vi "FunctDataMgr.Update Result Table Value.vi"(8 "error in (no error)":errorcluster, 11 "FunctDataMgr in":refnum<class "FunctDataMgr.lvclass">) -> (0 "error out":errorcluster, 3 "FunctDataMgr out":refnum<class "FunctDataMgr.lvclass">)   [LabVIEW 2018, in "FunctDataMgr.lvclass"]
uses:
  FunctDataMgr.lvclass
  FunctDataMgr.lvclass/FunctDataMgr.ctl
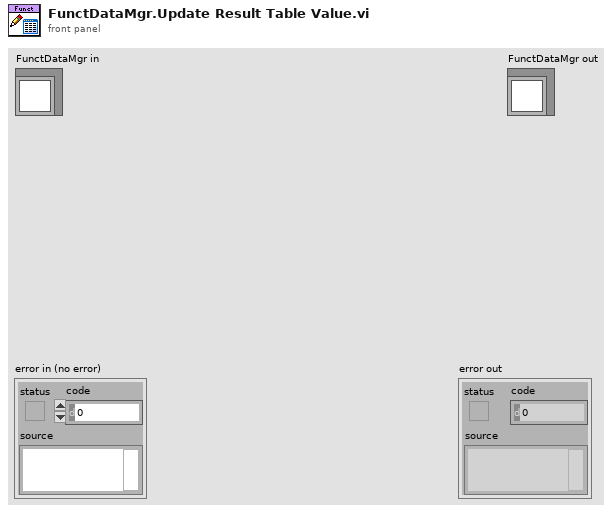
[diagram p1: front panel]
types:
  T1 = typedef "Report.Result FileDataObject.ctl" = cluster{"Cnt":i32, "Step":string, "Category":string, "Name":string, "Type":string, "File Name":string, "Time":string, "Path":path}
  T2 = typedef "Result.Numeric.ctl" = cluster{"Cnt":i32, "Step":string, "Category":string, "Name":string, "Value":dbl, "Units":string, "LimType":T3, "LL":dbl, "UL":dbl, "Status":T4, "Code":i32, "Desc":string, "Time":timestamp}
  T3 = typedef "Result.Limit Type.ctl" = enum16{"None", "EQ", "NE", "GT", "LT", "GE", "LE", "GTLT", "GELE", "GELT", "GTLE", "LTGT", "LEGE", "LEGT", "LTGE", "Contains", "NotContains"}
  T4 = typedef "Result.Measurement and Attribute Item Status.ctl" = i32
  T5 = typedef "Result.Attribute.ctl" = cluster{"Cnt":i32, "Step":string, "Category":string, "Name":string, "Value":string, "Status":T4, "Code":i32, "Desc":string, "Time":timestamp}
  T6 = typedef "Result.Measurement Item.ctl" = cluster{"Cnt":i32, "Step":string, "Category":string, "Name":string, "Value":string, "Units":string, "LimType":string, "LL":string, "UL":string, "Status":T4, "Code":i32, "Desc":string, "Time":timestamp}
  T7 = typedef "Result.Results Table Record.ctl" = cluster{"Cnt":i32, "Step":string, "Category":string, "Name":string, "Value":string, "Units":string, "LimType":string, "LL":string, "UL":string, "Status":string, "Status Color":u32, "Code":i32, "Desc":string}
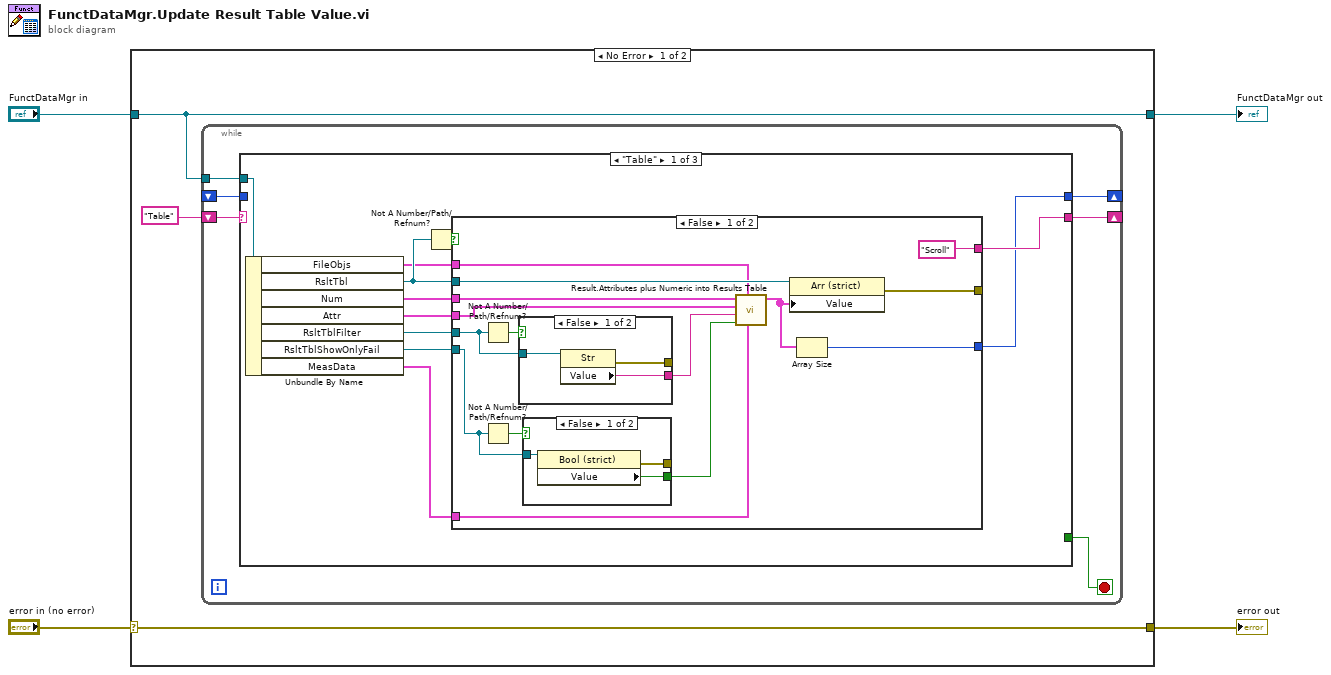
[diagram p0: block diagram]
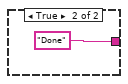
[diagram p4: hidden frame]
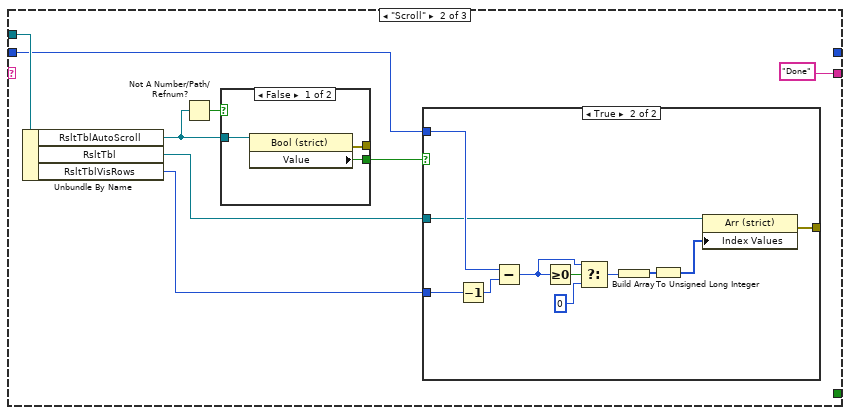
[diagram p5: hidden frame]
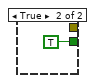
[diagram p7: hidden frame]
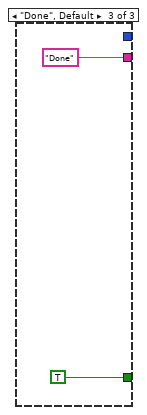
[diagram p8: hidden frame]
diagram:
  n1 = case shown="No Error" "error in (no error)" {
    selector: "error in (no error)" -> [w7 w73]
    tunnel: [w7 w73] -> w3
    tunnel: [w6 w72] -> w1
    tunnel: "FunctDataMgr in" -> [w6 w72]
    frame No Error {
      n2 = while {
        tunnel: w6 -> [w13]
        shift-right: [w10] -> _
        shift-left: "Table" -> [w12]
        shift-right: [w9] -> _
        shift-left: _ -> [w8]
        stop <- w11 stop-if-true
        n3 = case shown="\"Table\"" w12 {
          tunnel: w13 -> [w24 w54 _]
          tunnel: [_ _ TRUE] -> w11
          tunnel: [w21 "Done" "Done"] -> w10
          tunnel: [w16 _ _] -> w9
          tunnel: w8 -> [_ w50 _]
          frame "Table" {
            n4 = Unbundle By Name(w24) -> ("FileObjs"=w14:T1[], "RsltTbl"=w23:refnum<vi>, "Num"=w20:T2[], "Attr"=w19:T5[], "RsltTblFilter"=w18:refnum<vi>, "RsltTblShowOnlyFail"=w17:refnum<vi>, "MeasData"=w15:T6[])
            n5 = Not A Number/Path/Refnum?(number/path/refnum=w23) -> (NaN/Path/Refnum?=w22:bool)
            n6 = case shown="False" w22 {
              tunnel: w23 -> [w39 _]
              tunnel: [w38 _] -> _
              tunnel: ["Scroll" "Done"] -> w21
              tunnel: w20 -> [w36 _]
              tunnel: w19 -> [w35 _]
              tunnel: w18 -> [w34 _]
              tunnel: w17 -> [w30 _]
              tunnel: [w27 _] -> w16
              tunnel: w15 -> [w26 _]
              tunnel: w14 -> [w25 _]
              frame False {
                n7 = Not A Number/Path/Refnum?(number/path/refnum=w34) -> (NaN/Path/Refnum?=w33:bool)
                n8 = Not A Number/Path/Refnum?(number/path/refnum=w30) -> (NaN/Path/Refnum?=w31:bool)
                n9 = case shown="False" w33 {
                  tunnel: w34 -> [w45 _]
                  tunnel: [w44 _] -> _
                  tunnel: [w43 _] -> w32
                  frame False {
                    n10 = property class="Str"(reference=w45) -> (error out=w44:errorcluster, "Value"=w43:string)  [unwired: 1 in, 1 out]
                  }
                  frame True {
                  }
                }
                n11 = case shown="False" w31 {
                  tunnel: w30 -> [w42 _]
                  tunnel: [w41 _] -> _
                  tunnel: [w40 _] -> w29
                  frame False {
                    n12 = property class="Bool (strict)"(reference=w42) -> (error out=w41:errorcluster, "Value"=w40:bool)  [unwired: 1 in, 1 out]
                  }
                  frame True {
                  }
                }
                n13 = call "Result.Attributes plus Numeric into Results Table.vi"("Meas"=w26, "File Data Objs"=w25, "Show Only Failures"=w29, "Filter"=w32, "Attribute Data"=w35, "Numeric Data"=w36) -> ("Results Table"=w28:T7[])  [unwired: 5 in]
                n14 = property class="Arr (strict)"(reference=w39, "Value"=w28) -> (error out=w38:errorcluster)  [unwired: 1 in, 1 out]
                n15 = Array Size(array=w28) -> (size(s)=w27:i32)
              }
              frame True {
              }
            }
          }
          frame "Scroll" {
            n16 = Unbundle By Name(w54) -> ("RsltTblAutoScroll"=w53:refnum<vi>, "RsltTbl"=w47:refnum<vi>, "RsltTblVisRows"=w48:i32)
            n17 = Not A Number/Path/Refnum?(number/path/refnum=w53) -> (NaN/Path/Refnum?=w52:bool)
            n18 = case shown="False" w52 {
              tunnel: w53 -> [w68 _]
              tunnel: [w67 TRUE] -> w49
              tunnel: [w66 _] -> _
              frame False {
                n19 = property class="Bool (strict)"(reference=w68) -> (error out=w66:errorcluster, "Value"=w67:bool)  [unwired: 1 in, 1 out]
              }
              frame True {
              }
            }
            n20 = case shown="True" w49 {
              tunnel: w50 -> [_ w60]
              tunnel: w48 -> [_ w59]
              tunnel: w47 -> [_ w58]
              tunnel: [_ w56] -> _
              frame False {
              }
              frame True {
                n21 = Decrement(x=w59) -> (x-1=w61:i32)
                n22 = Subtract(x=w60, y=w61) -> (x-y=w55:i32)
                n23 = Greater Or Equal To 0?(x=w55) -> (x >= 0?=w62:bool)
                n24 = Select(t=w55, s=w62, f=0) -> (s? t:f=w64:i32)
                n25 = Build Array(w64) -> (w65:i32[])
                n26 = To Unsigned Long Integer(number=w65) -> (unsigned 32bit integer=w57:u32[])
                n27 = property class="Arr (strict)"(reference=w58, "Index Values"=w57) -> (error out=w56:errorcluster)  [unwired: 1 in, 1 out]
              }
            }
          }
          frame "Done", Default {
          }
        }
      }
    }
    frame Error {
    }
  }
  "error out" <- w3
  "FunctDataMgr out" <- w1
